vi "CRYSave Excel.vi"(0 "error in (no error)":errorcluster, 2 "FilePath":string, 3 "Excel._Workbook":refnum<k7>) -> (7 "error out":errorcluster)   [LabVIEW 2013]
doc: "This VI opens Excel by creating an Automation Refnum for the Excel.Application object. Next it sets the \"Visible\" property to True/False depending on the Visible input."
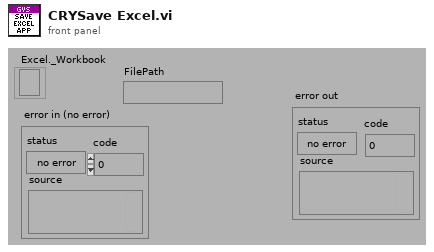
[diagram p1: front panel]
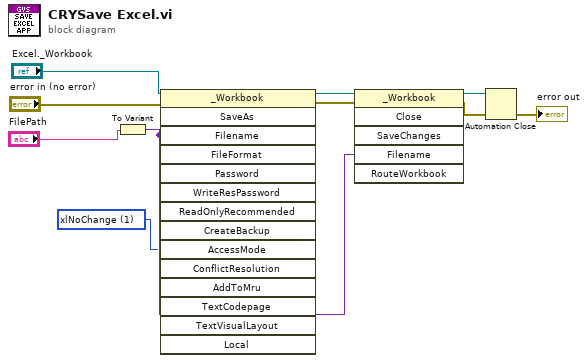
[diagram p0: block diagram]
diagram:
  w4 = 1 items=["xlExclusive"=3, "xlNoChange"=1, "xlShared"=2] ("AccessMode")
  n1 = To Variant(anything="FilePath") -> (Variant=w7:variant)
  n2 = invoke class="_Workbook" method="SaveAs"(reference="Excel._Workbook", error in="error in (no error)", "Filename"=w7, "AccessMode"=w4) -> (reference out=w5:refnum<k7>, error out=w6:errorcluster)  [unwired: 11 in, 13 out]
  n3 = invoke class="_Workbook" method="Close"(reference=w5, error in=w6, "Filename"=w7) -> (reference out=w3:refnum<k7>, error out=w2:errorcluster)  [unwired: 3 in, 4 out]
  n4 = Automation Close(3:w2, 5:w3) -> (0:→"error out":errorcluster)
